vi "cypher read value_MFP3D_Lucy.vi"(11 "Input":u16(ring) items=["XSensor", "YSensor", "ZSensor", "InA", "InB", "InFast", "In_Amplitude1", "In_Amplitude2", "In_Phase1", "In_Phase2", "PiezoX", "PiezoY", "PiezoZ", "OutA", "OutB", "OutC", "DDS_Frequency1", "DDS_Frequency2", "DDS_Amplitude1", "DDS_Amplitude2", "DDS_DCOffset", "Laser_Sum", "Laser_Difference", "Laser_Lateral", "XLVDT Sensitivity", "YLVDT Sensitivity", "XLVDT Offset", "YLVDT Offset", "PIDSLoop.0.Setpoint", "PIDSLoop.1.Setpoint"]) -> (3 "Result":dbl format="%#_5p")   [LabVIEW 2019]
doc: "This Vi can help read out the parameteres, signal channels in AFM."
panel:
  out "error out":errorcluster
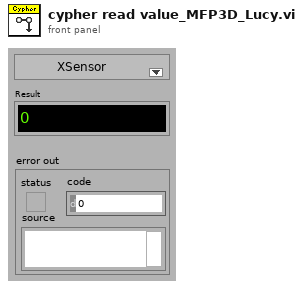
[diagram p1: front panel]
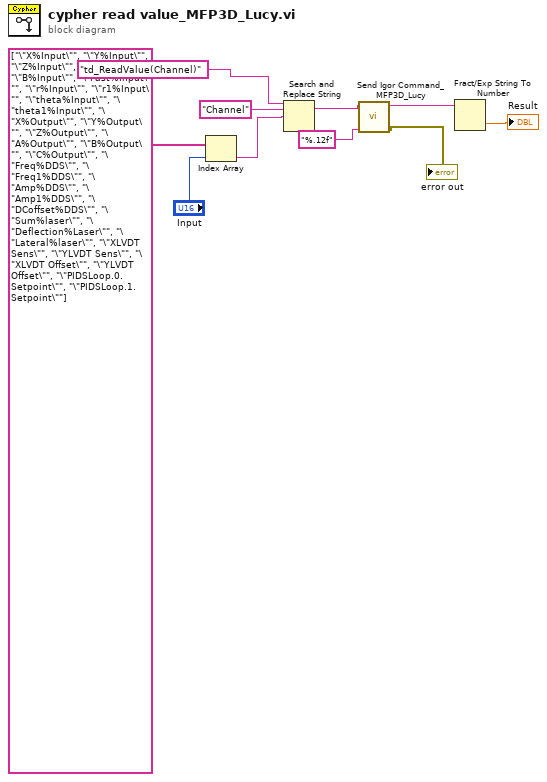
[diagram p0: block diagram]
diagram:
  n1 = Index Array(array=string[] ["\"X%Input\"", "\"Y%Input\"", "\"Z%Input\"", "\"A%Input\"", "\"B%Input\"", "\"Fast%Input\"", "\"r%Input\"", "\"r1%Input\"", "\"theta%Input\"", "\"theta1%Input\"", "\"X%Output\"", "\"Y%Output\"", "\"Z%Output\"", "\"A%Output\"", "\"B%Output\"", "\"C%Output\"", "\"Freq%DDS\"", "\"Freq1%DDS\"", "\"Amp%DDS\"", "\"Amp1%DDS\"", "\"DCoffset%DDS\"", "\"Sum%laser\"", "\"Deflection%Laser\"", "\"Lateral%laser\"", "\"XLVDT Sens\"", "\"YLVDT Sens\"", "\"XLVDT Offset\"", "\"YLVDT Offset\"", "\"PIDSLoop.0.Setpoint\"", "\"PIDSLoop.1.Setpoint\""], index="Input") -> (element=w8:string)
  n2 = Search and Replace String(input string="td_ReadValue(Channel)", search string="Channel", replace string=w8) -> (result string=w4:string)  [unwired: 1 in, 7 out]
  n3 = call "Send Igor Command_MFP3D_Lucy.vi"("Command"=w4, "Expected output Format"="%.12f") -> ("results"=w1:string, "error out"=→"error out":errorcluster)  [unwired: 6 in, 1 out]
  n4 = Fract/Exp String To Number(string=w1) -> (number=→"Result":dbl)  [unwired: 4 out]
